vi "Dashboard Main.vi"() -> ()   [LabVIEW 2014]
uses:
  <vilib>/event_ctls.llb/eventvkey.ctl
  <vilib>/Utility/config.llb/NI_LVConfig.lvlib
  <vilib>/Rock Robotics/WPI/Dashboard/WPI_DashboardLogging Global.vi
  <vilib>/Rock Robotics/Network Tables/SD Read Number.vi
  <vilib>/Rock Robotics/Network Tables/SD Write Number.vi
  <vilib>/Utility/config.llb/Write Key (I32).vi
  <vilib>/Utility/config.llb/Write Key (String).vi
  <vilib>/Rock Robotics/Network Tables/SD Read String.vi
  <vilib>/Rock Robotics/Network Tables/SD Read Boolean.vi
  <vilib>/Rock Robotics/Network Tables/SD Write Boolean.vi
panel:
  in  "TCP":refnum<k5>
  in  "Rec Mode":enum32{"Stop", "Record", "Playback"}(radio)
  in  "Vision":u16(ring) items=["Camera Off", "USB Camera SW", "USB Camera HW", "IP Camera"]
  out "Camera IP":string
  out "Image Message":string="Timeout in Camera Communications"
  in  "Dashboard Tab":T1(tab)
  in  "Camera Guide Position":dbl(slide)=216.05839416058393 scale=0.0..320.0
  in  "Camera Settings":T2={"Frame Rate"=30, "Compression"=30, "Size"=1} {"Frame Rate" scale=1.0..30.0; "Size" items=["640x480", "320x240", "160x120"]}
  out "MotorChart R":cluster{"Numeric":dbl, "Numeric":dbl}(graph)
  out "MotorChart L":T3(graph)
  out "MotorSliders R":cluster{"MotorSlide1":dbl, "MotorSlide2":dbl} {"MotorSlide2" scale=-1.0..1.0 scale format="%#_2e"; "MotorSlide1" scale=-1.0..1.0 scale format="%#_2e"}
  out "MotorSliders L":T4 {"MotorSlide4 2" scale=0.0..14.0 scale format="%#_2e"; "MotorSlide2" scale=-1.0..1.0 scale format="%#_2e"; "MotorSlide1" scale=-1.0..1.0 scale format="%#_2e"}
  out "JS1 Z":dbl(slide) scale=-1.0..1.0 scale format="%#_2e"
  out "JS1 Graph":cluster{"X":dbl, "Y":dbl}[](graph)
  out "JS1 Buttons":T5
  out "JS2 Z":dbl(slide) scale=-1.0..1.0 scale format="%#_2e"
  out "JS2 Graph":cluster{"X":dbl, "Y":dbl}[](graph)
  out "JS2 Buttons":T5
  out "Mode":T6(ring)=enum."Auto Disabled"
  in  "DB Camera Config":bool
  out "fps":dbl format="%#.1g"
  out "Mbps":dbl format="%#.1g"
  out "Mbps 2":bool
  in  "FastAuto?":bool
  in  "AutoStackRamp":bool
  out "Current Auto":dbl
  out "Auto/String 3":string caption="DB/String 3"
  out "Auto/String 2":string caption="DB/String 2"
  out "Auto/String 1":string caption="DB/String 1"
  out "Auto/String 0":string caption="Auto"
  out "Elev. Current":dbl
  out "Can\n  Auto\n  Stack":bool
  out "PID State":T7(ring)
  in  "Training Mode Threshold":dbl=0.8
  out "Drive Mode":bool
  out "Gyro":dbl(knob) scale=0.0..360.0
  in  "Halo Sensitivity":dbl=0.7 min=0.0 max=1.0 step=0.01 format="%.2f"
  out "Encoder Left":dbl
  out "Encoder Right":dbl
  out "Training Enabled":bool
  out "Auto Stack State":T8(ring)
  out "Gripper":bool
  out "Gripper 2":bool
  out "Elev. Target":dbl
  in  "Test Slider":dbl(slide) scale=0.0..100.0 scale format="%#_3g"
  in  "On/Off":bool caption="Solenoid"
  in  "Test Name":u16(ring) items=["Select the test to run...", "Example Test", "-------------------------------", "List of tests is built in robot code.", "Replace with your own automated tests."]
  in  "Test Tree":string(tree)
  in  "Motor":cluster{"Value":dbl, "Enable":bool} {"Value" scale=-1.0..1.0 scale format="%#_3g"}
  out "Progress":T9 {"Test Progress" scale=0.0..100.0}
  in  "Rev/Fwd":cluster{"Forward":bool, "Reverse":bool}
  in  "Test Ring":u16(ring) items=["Monochrome", "Color"]
  in  "Listbox":i32(listbox)
  out "Tree":string(tree)
  out "Camera Image":T10(plugin-control)
  out "Boolean":bool
  # "Left"
  # "Front"
  # "Right"
  # "Battery"
  # "AUTO STACK"
  # "0 - TOTE+CONTAINER\n1 - DRIVESTRAIGHT FROM STARTING AREA\n2 - DRIVESTRAIGHT FROM VOLDEMORT\n3 - 2 CONTAINER + LEFT TURN\n4 - 2 CONTAINER + RIGHT TURN\n5 - STOP_ALL\n6 - TAPE MEASURE\n7 - TOTE TO FEEDER - SHORT\n8 - TOTE TO FEEDER - LONG\n9 - CAN BURGLAR"
  # "Hold BACK button on \nJoystick 1 to switch"
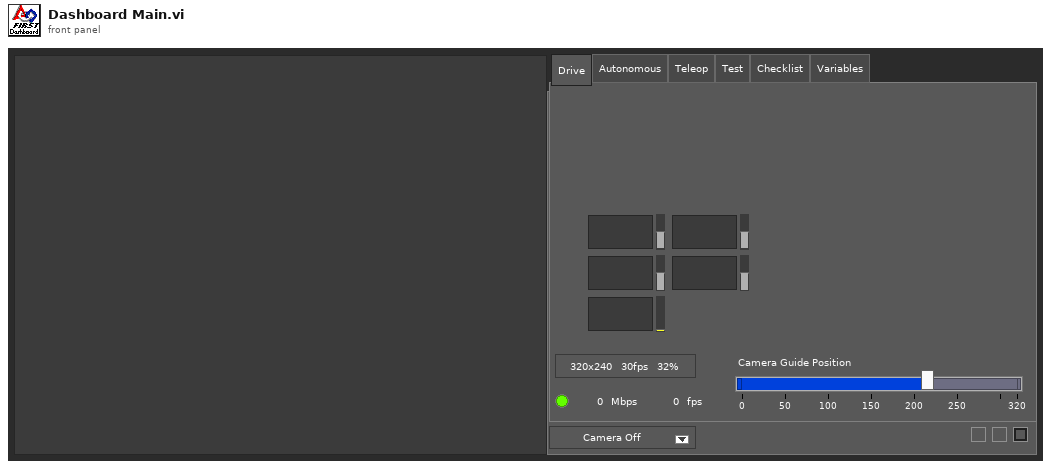
[diagram p1: front panel]
types:
  T1 = enum32{"Drive", "Autonomous", "Teleop", "Test", "Checklist", "Variables"}
  T2 = cluster{"Frame Rate":i32, "Compression":i32, "Size":u16}
  T3 = cluster{"Numeric":dbl, "Numeric":dbl, "Battery V":dbl}
  T4 = cluster{"MotorSlide1":dbl, "MotorSlide2":dbl, "MotorSlide4 2":dbl}
  T5 = cluster{bool, bool, bool, bool, bool, bool, bool, bool, bool, bool, bool, bool}
  T6 = enum8{"Tele-Op Disabled", "Tele-Op Enabled", "Auto Disabled", "Auto Enabled", "Test Disabled", "Test Enabled", "Disconnected", "No Code", "E-Stop"}
  T7 = enum16{"ResetForward", "ResetBack", "PIDControl", "ManualControl", "ZeroEncoderAndTarget", "AutoStack"}
  T8 = enum16{"Disabled", "Initialize", "CalcNewTarget", "Moving", "OpenArm", "CloseArm", "Reset"}
  T9 = cluster{"Test Progress":u8, "Test Progress Text":string}
  T10 = typedef "IMAQ Image.ctl" = refnum<image>
  T11 = enum32{"Drive", "Basic", "Custom", "Test", "Checklist", "Variables"}
  T12 = typedef "Image Type" = u32
  T13 = cluster{"Camera Image":refnum<vi>, "Dashboard Tab":refnum<vi>, "Boolean":refnum<vi>, "Vision":refnum<vi>, "Rec Mode":refnum<vi>, "Test Slider":refnum<vi>, "On/Off ":refnum<vi>, "Test Ring":refnum<vi>, "Rev/Fwd":refnum<vi>, "Test Name":refnum<vi>, "Motor":refnum<vi>, "Progress":refnum<vi>, "CheckList":refnum<vi>, "Tree":refnum<vi>, "Test Tree":refnum<vi>}
  T14 = cluster{"Error Strings":string, "Disable Counts":cluster{u16, u16}, "Rail Faults":cluster{u16, u16, u16}, "Robot IP":string, "DB Mode":u8, "Event Info":cluster{"Name":string, "Type":u8, "Number":u16, "Replay":u8}, "Camera Addr":string}
  T15 = cluster{"Storage":cluster{"Disk Free":u64, "RAM Block":u32, "RAM free":u32}, "CPU Utilization":cluster{"CPU % ISR":sgl, "CPU % Time Crit":sgl, "CPU % Timed Str":sgl, "CPU % High":sgl, "CPU % Above":sgl, "CPU % Normal":sgl, "CPU % Low":sgl}, "CAN":cluster{"% Bus Utilization":sgl, "Bus Off Cnt":u32, "TX_FIFO Full Cnt":u32, "Receive Error Cnt":u8, "Transmit Error Cnt":u8}, "HID":cluster{"HID Outputs":u32, "Rumble Low":u16, "Rumble High":u16}[]}
  T16 = cluster{"Status bits":cluster{"Test Mode":bool, "Autonomous":bool, "Enabled":bool, "Code Start":bool, "Brownout":bool, "Reserved 2":bool, "Reserved 3":bool, "E-Stop":bool}, "Code Trace":cluster{"Disabled":bool, "TeleOp":bool, "Auto":bool, "Test":bool}, "Controller Type":enum16{"unknown", "cRIO", "roboRio"}, "Code?":enum16{"unknown", "noCode", "code"}, "Battery V":dbl}
  T17 = cluster{"Control Bits":cluster{"TestMode":bool, "Autonomous":bool, "Enabled":bool, "FMS Present":bool, bool, bool, bool, "E-Stop":bool}, "Team Station ":u8, "Countdown":sgl, "Joystick Values":cluster{"Axes":dbl[], "Buttons":bool[], "POVs":i16[]}[]}
  T18 = cluster{"Axes":dbl[], "Buttons":bool[], "POVs":i16[]}[]
  T19 = cluster{"Axes":dbl[], "Buttons":bool[], "POVs":i16[]}
  T20 = cluster{"Buttons[0]":bool, "Buttons[1]":bool, "Buttons[2]":bool, "Buttons[3]":bool, "Buttons[4]":bool, "Buttons[5]":bool, "Buttons[6]":bool, "Buttons[7]":bool, "Buttons[8]":bool, "Buttons[9]":bool, "Buttons[10]":bool, "Buttons[11]":bool}
  T21 = typedef "NI_LVConfig.lvlib/Config Data RefNum.ctl" = refnum<k1>
  T22 = cluster{"Operation":enum16{"Update", "Clear"}, "Color Box":u32}[]
  T23 = typedef "eventvkey.ctl" = enum16{"ASCII", "Enter", "Return", "Shift", "Ctrl", "Alt", "Cmd", "Opt", "Caps", "NumLock", "Clear", "Break", "Up", "Down", "Left", "Right", "Insert", "Delete", "Home", "End", "PageUp", "PageDown", "Escape", "Help", "Pause", "ScrollLock", "F1", "F2", "F3", "F4", "F5", "F6", "F7", "F8", "F9", "F10", "F11", "F12", "F13", "F14", "F15", "F16", "F17", "F18", "F19", "F20", "F21", "F22", "F23", "F24", "Play", "VolumeUp", "VolumeDown", "Mute", "Two Byte Char"}
  T24 = cluster{"Image Size":bool, "Image Type":bool, "Pixel Value":bool, "ROI Information":bool, "Zoom Factor":bool}
  T25 = enum8{"Enabled", "Disabled", "Disabled and Grayed Out"}
  T26 = cluster{"Operation":enum16{"Update", "Clear"}, "Color Box":u32}
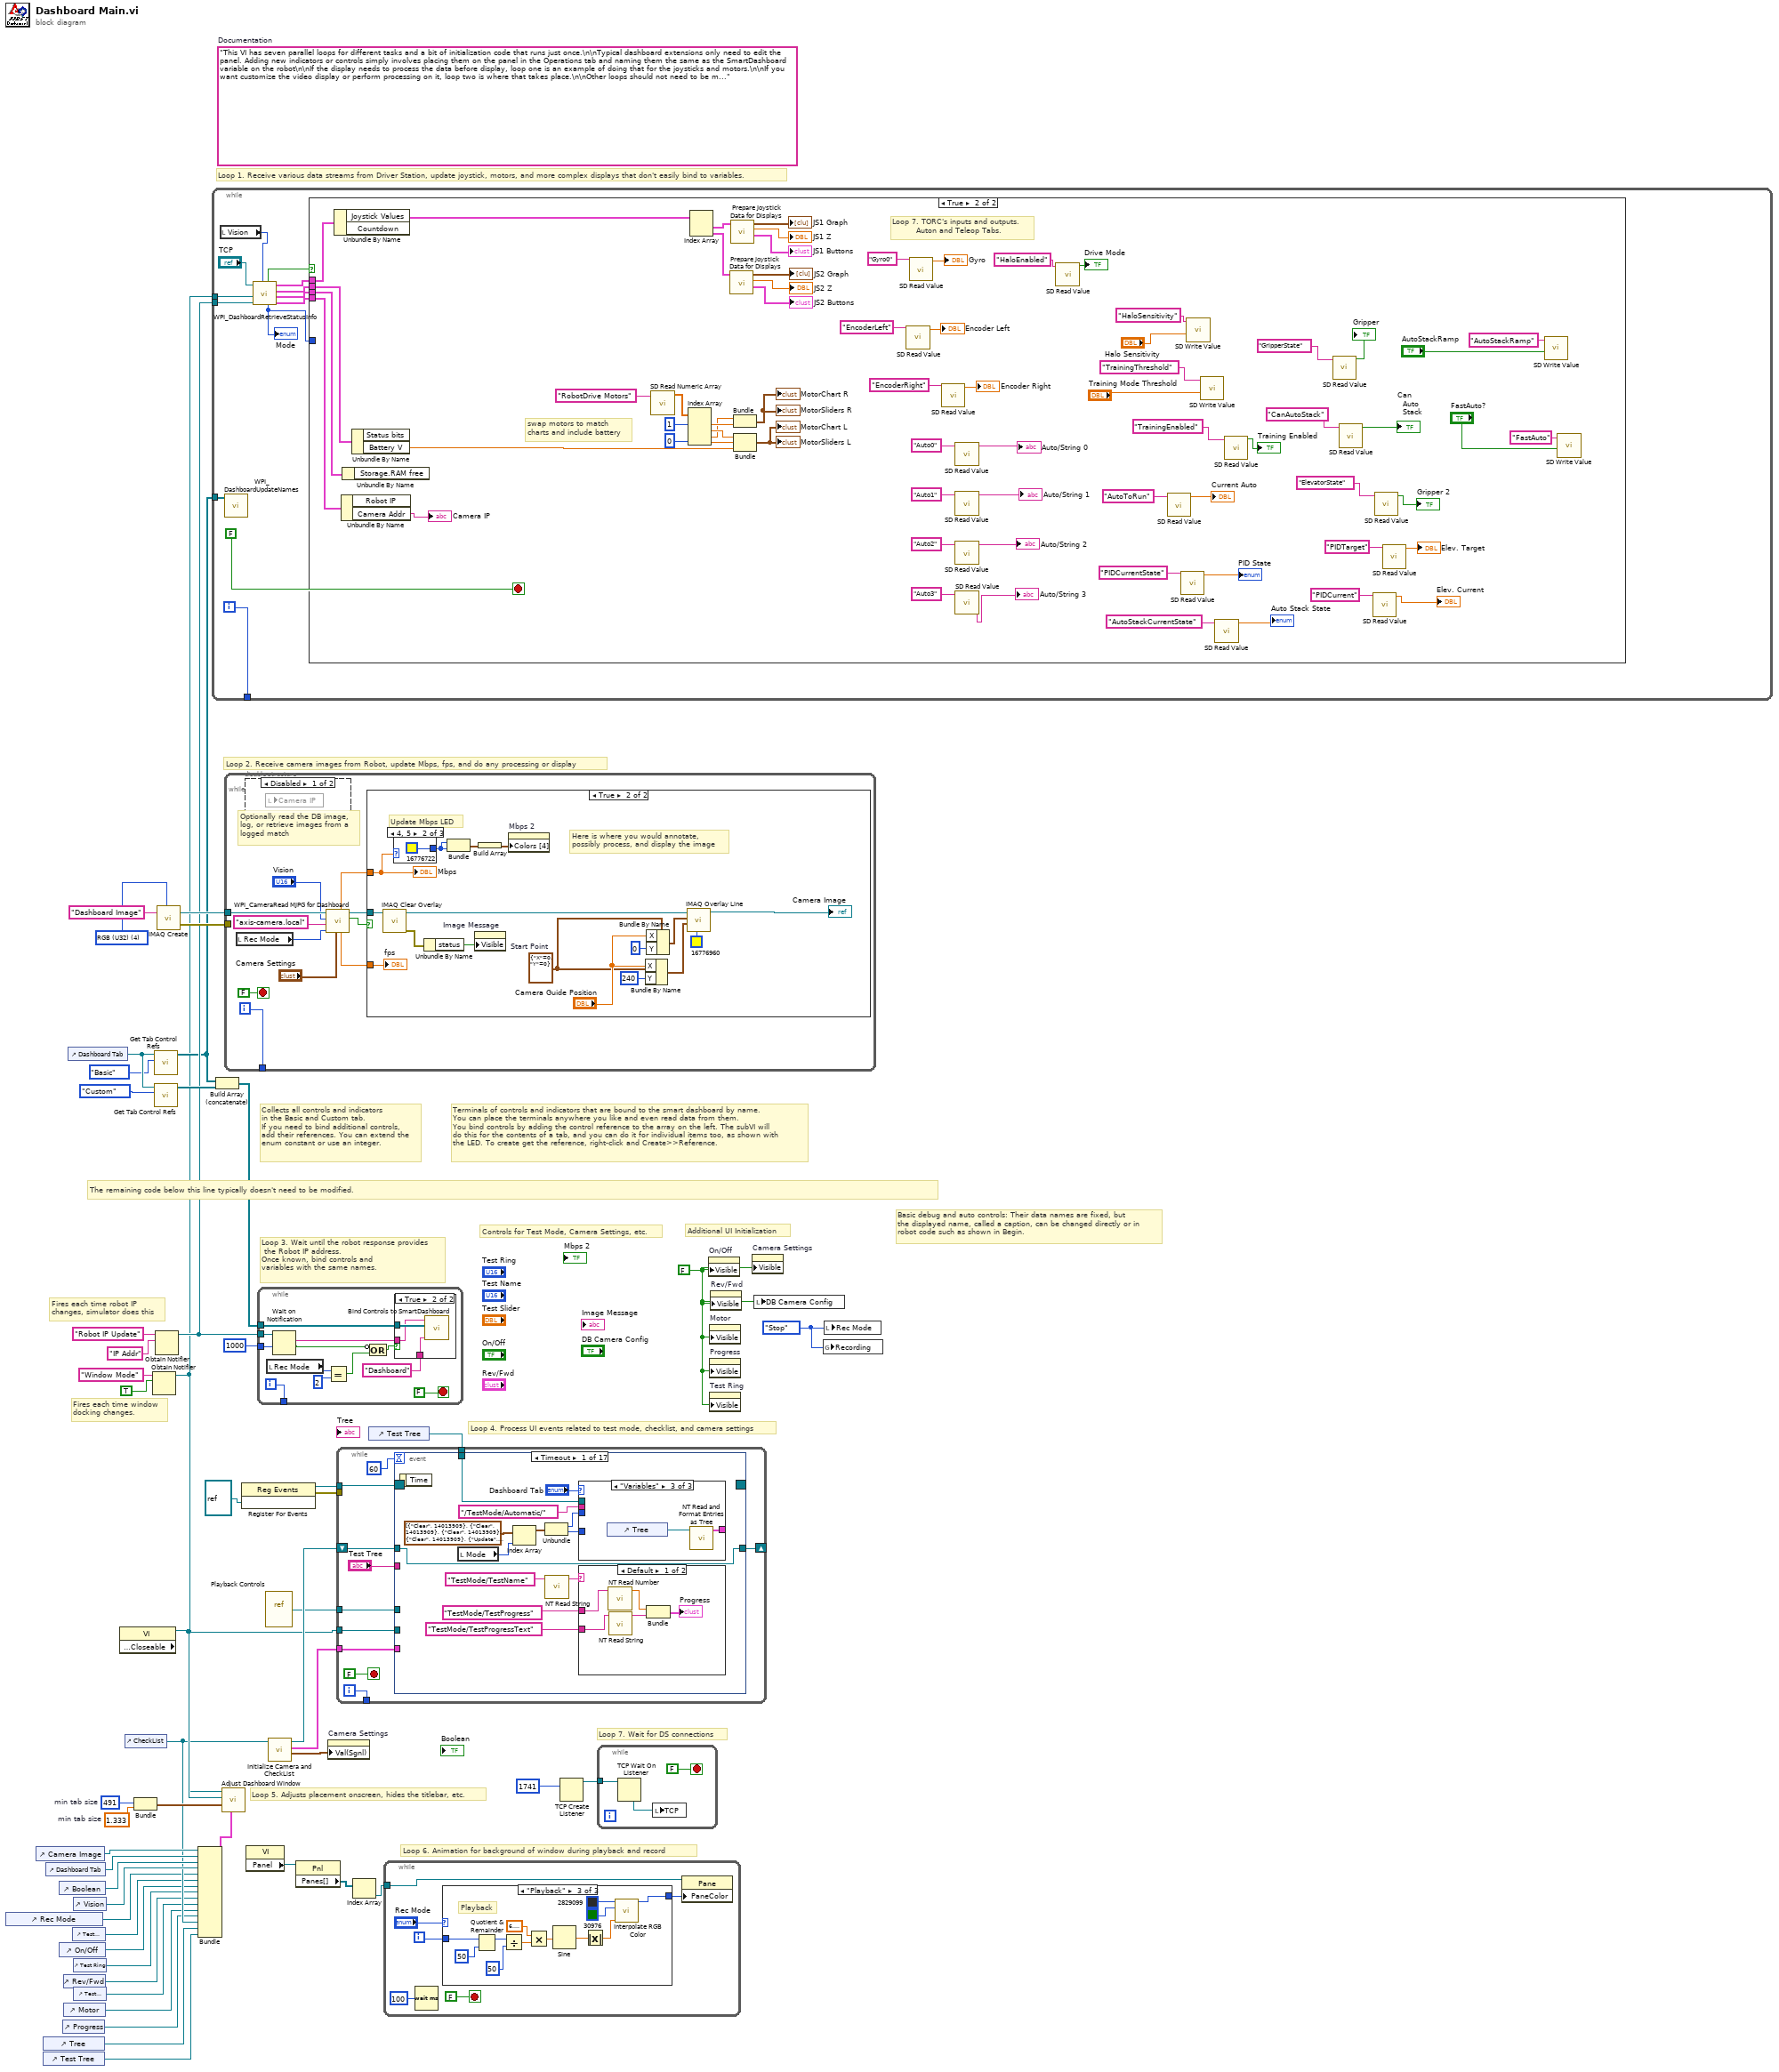
[diagram p0: block diagram]
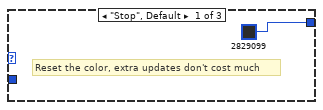
[diagram p3: hidden frame]
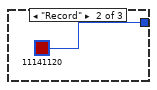
[diagram p4: hidden frame]
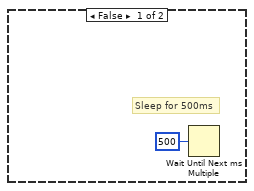
[diagram p7: hidden frame]
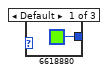
[diagram p8: hidden frame]
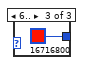
[diagram p9: hidden frame]
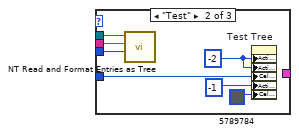
[diagram p11: hidden frame]
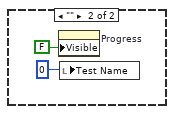
[diagram p12: hidden frame]
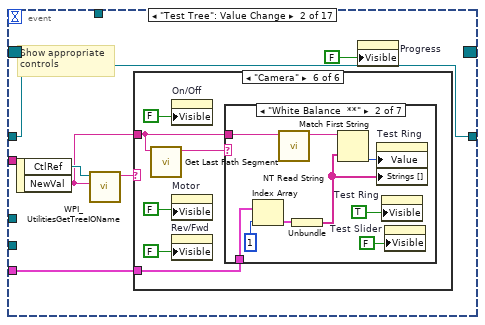
[diagram p13: hidden frame]
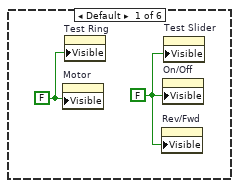
[diagram p14: hidden frame]
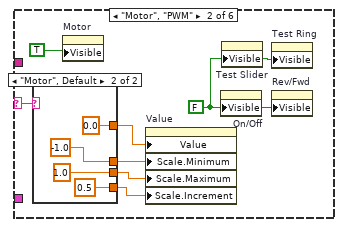
[diagram p15: hidden frame]
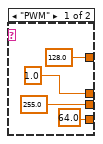
[diagram p16: hidden frame]
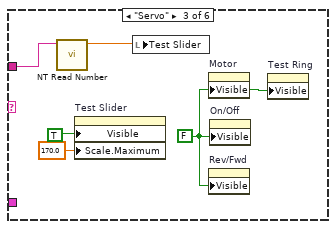
[diagram p17: hidden frame]
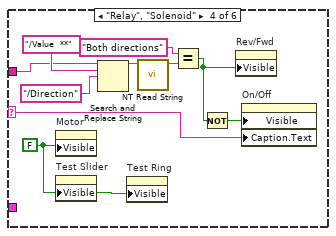
[diagram p18: hidden frame]
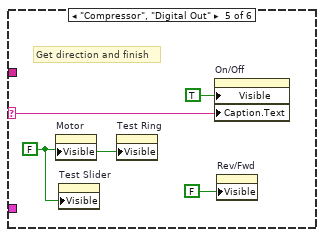
[diagram p19: hidden frame]
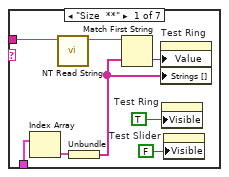
[diagram p20: hidden frame]
diagram:
  w24 = 491  # min tab size
  w23 = 1.333  # min tab size
  w32 = enum32{"Stop", "Record", "Playback"}."Stop" ("Rec Mode")
  w6 = FALSE ("Visible")
  (unwired) "This VI has seven parallel loops for different tasks and a bit of initialization code that runs just once.\n\nTypical dashboard extensions only need to edit the panel. Adding new indicators or controls simply involves placing them on the panel in the Operations tab and naming them the same as the SmartDashboard variable on the robot\n\nIf the display needs to process the data before display, loop one is an example of doing that for the joysticks and motors.\n\nIf you want customize the video display or perform processing on it, loop two is where that takes place.\n\nOther loops should not need to be modified. They are pretty standard, and document the task they perform."  # Documentation
  w52 = T12 4 items=["Grayscale (U8)", "Grayscale (I16)", "Grayscale (SGL)", "Complex (CSG)", "RGB (U32)", "HSL (U32)", "RGB (U64)"] ("Image Type")
  # "Loop 7. Wait for DS connections"
  # "Basic debug and auto controls: Their data names are fixed, but\nthe displayed name, called a caption, can be changed directly or in\nrobot code such as shown in Begin."
  # "Controls for Test Mode, Camera Settings, etc."
  # "Additional UI Initialization"
  # "Loop 6. Animation for background of window during playback and record"
  # "Fires each time robot IP\nchanges, simulator does this"
  # "Fires each time window\ndocking changes."
  # "Collects all controls and indicators\nin the Basic and Custom tab.\nIf you need to bind additional controls,\nadd their references. You can extend the\nenum constant or use an integer."
  # "The remaining code below this line typically doesn't need to be modified."
  # "Loop 4. Process UI events related to test mode, checklist, and camera settings"
  # "Terminals of controls and indicators that are bound to the smart dashboard by name.\nYou can place the terminals anywhere you like and even read data from them.\nYou bind controls by adding the control reference to the array on the left. The subVI will\ndo this for the contents of a tab, and you can do it for individual items too, as shown with\nthe LED. To create get the reference, right-click and Create>>Reference."
  # "Loop 3. Wait until the robot response provides\n the Robot IP address.\nOnce known, bind controls and\nvariables with the same names."
  # "Loop 5. Adjusts placement onscreen, hides the titlebar, etc."
  # "Loop 1. Receive various data streams from Driver Station, update joystick, motors, and more complex displays that don't easily bind to variables."
  # "Loop 2. Receive camera images from Robot, update Mbps, fps, and do any processing or display"
  n1 = control-ref of="Rec Mode"() -> (w12:refnum<vi>)
  n2 = control-ref of="Camera Image"() -> (w27:refnum<vi>)
  n3 = control-ref of="Tree"() -> (w16:refnum<vi>)
  n4 = control-ref of="Test Tree"() -> (w15:refnum<vi>)
  n5 = control-ref of="Dashboard Tab"() -> (w26:refnum<vi>)
  n6 = control-ref of="Boolean"() -> (w21:refnum<vi>)
  n7 = control-ref of="On/Off"() -> (w10:refnum<vi>)
  n8 = control-ref of="Progress"() -> (w7:refnum<vi>)
  n9 = control-ref of="Rev/Fwd"() -> (w8:refnum<vi>)
  n10 = control-ref of="Motor"() -> (w13:refnum<vi>)
  n11 = control-ref of="Dashboard Tab"() -> (w30:refnum<vi>)
  n12 = control-ref of="Test Slider"() -> (w11:refnum<vi>)
  n13 = control-ref of="Vision"() -> (w25:refnum<vi>)
  n14 = control-ref of="Test Ring"() -> (w9:refnum<vi>)
  n15 = control-ref of="Test Name"() -> (w14:refnum<vi>)
  n16 = property class="VI" props=["Front Panel.Closeable"]() -> (reference out=w31:refnum<vi>)  [unwired: 2 in, 2 out]
  n17 = control-ref of="CheckList"() -> (w17:refnum<vi>)
  n18 = Bundle("min tab size"=w24, "min tab size"=w23) -> (w22:cluster{"min tab size":i32, "min tab size":dbl})  [unwired: 1 in]
  n19 = Obtain Notifier(name (unnamed)="Window Mode", notification data type=TRUE) -> (notifier out=w3:refnum<notifier>)  [unwired: 2 in, 2 out]
  n20 = call <vilib>:"Get Tab Control Refs.vi"("Page Index"=T11."Basic" ("Dashboard Tab"), "TabControl in"=w30) -> ("ControlsOnPage"=w4:refnum<vi>[])  [unwired: 9 in]
  n21 = call <vilib>:"Get Tab Control Refs.vi"("Page Index"=T11."Custom" ("Dashboard Tab"), "TabControl in"=w30) -> ("ControlsOnPage"=w29:refnum<vi>[])  [unwired: 9 in]
  n22 = Obtain Notifier(name (unnamed)="Robot IP Update", notification data type="IP Addr" ("name (unnamed)")) -> (notifier out=w5:refnum<notifier>)  [unwired: 2 in, 2 out]
  n23 = call "IMAQ Create"("Image Name"="Dashboard Image", "Image Type"=w52) -> ("New Image"=w50:T10, "error out"=w49:errorcluster)  [unwired: 2 in, 1 out]
  n24 = Bundle("Camera Image"=w27, "Dashboard Tab"=w26, "Boolean"=w21, "Vision"=w25, "Rec Mode"=w12, "Test Slider"=w11, "On/Off"=w10, "Test Ring"=w9, "Rev/Fwd"=w8, "Test Name"=w14, "Motor"=w13, "Progress"=w7, "CheckList"=w17, "Tree"=w16, "Test Tree"=w15) -> (w18:T13)  [unwired: 1 in]
  n25 = while {
    tunnel: [w64] -> _
    tunnel: w5 -> [w63]
    tunnel: w4 -> [w62]
    tunnel: w3 -> [w59]
    i -> [w64]
    stop <- FALSE stop-if-true
    n26 = local read "Vision"() -> (w61:u16)
    n27 = call <vilib>:"WPI_DashboardUpdateNames.vi"("Controls on Tab"=w62) -> ()  [unwired: 11 in]
    n28 = call <vilib>:"WPI_DashboardRetrieveStatusInfo.vi"("Vision"=w61, "Binding Refnum"=w63, "Window Mode Notifier"=w59, "TCP Cnx"="TCP") -> ("Power and Errors"=w55:T14, "Robot Metrics"=w56:T15, "Status Info"=w57:T16, "Control Info"=w58:T17, "Robot Mode"=w54:T6, "Process?"=w53:bool)  [unwired: 2 in]
    "Mode" <- w54
    n29 = case shown="True" w53 {
      tunnel: w57 -> [_ w132]
      tunnel: w56 -> [_ w131]
      tunnel: w58 -> [_ w130]
      tunnel: w55 -> [_ w129]
      tunnel: w54 -> [_ _]
      frame False {
      }
      frame True {
        # "Loop 7. TORC's inputs and outputs.\n         Auton and Teleop Tabs."
        # "swap motors to match\ncharts and include battery"
        n30 = Unbundle By Name(w130) -> ("Joystick Values"=w117:T18)  [unwired: 1 out]
        n31 = Unbundle By Name(w129) -> ("Camera Addr"=→"Camera IP":string)  [unwired: 1 out]
        n32 = Unbundle By Name(w131) -> ()  [unwired: 1 out]
        n33 = Unbundle By Name(w132) -> ("Battery V"=w118:dbl)  [unwired: 1 out]
        n34 = call <vilib>:"SD Read Numeric Array.vi"("Name"="RobotDrive Motors") -> ("Numeric Array"=w120:dbl[])  [unwired: 8 in, 2 out]
        n35 = Index Array(array=w120, index #1=1, index #4=0) -> (element #1=w124:dbl, element #2=w125:dbl, element #3=w123:dbl, element #4=w128:dbl)  [unwired: 2 in]
        n36 = Index Array(array=w117) -> (element #1=w116:T19, element #2=w111:T19)  [unwired: 2 in]
        n37 = call "Prepare Joystick Data for Displays.vi"("Joystick Values"=w111) -> ("Buttons"=→"JS2 Buttons":T20, "Z Axis"=→"JS2 Z":dbl, "Cartesian Data"=→"JS2 Graph":cluster{"X axis":dbl, "X axis":dbl}[])  [unwired: 8 in]
        n38 = call "Prepare Joystick Data for Displays.vi"("Joystick Values"=w116) -> ("Buttons"=→"JS1 Buttons":T20, "Z Axis"=→"JS1 Z":dbl, "Cartesian Data"=→"JS1 Graph":cluster{"X axis":dbl, "X axis":dbl}[])  [unwired: 8 in]
        n39 = Bundle("Numeric"=w123, "Numeric"=w124) -> (→"MotorChart R" →"MotorSliders R":cluster{"Numeric":dbl, "Numeric":dbl})  [unwired: 1 in]
        n40 = Bundle("Numeric"=w125, "Numeric"=w128, "Battery V"=w118) -> (→"MotorChart L" →"MotorSliders L":T3)  [unwired: 1 in]
        n41 = call-poly <vilib>:"SD Read Value.vi"("Name"="EncoderLeft") -> ("Numeric"=→"Encoder Left":dbl)  [unwired: 8 in, 2 out]
        n42 = call-poly <vilib>:"SD Read Value.vi"("Name"="Gyro0") -> ("Numeric"=→"Gyro":dbl)  [unwired: 8 in, 2 out]
        n43 = call-poly <vilib>:"SD Read Value.vi"("Name"="EncoderRight") -> ("Numeric"=→"Encoder Right":dbl)  [unwired: 8 in, 2 out]
        n44 = call-poly <vilib>:"SD Read Value.vi"("Name"="Auto0") -> ("String"=→"Auto/String 0":string)  [unwired: 8 in, 2 out]
        n45 = call-poly <vilib>:"SD Read Value.vi"("Name"="Auto1") -> ("String"=→"Auto/String 1":string)  [unwired: 8 in, 2 out]
        n46 = call-poly <vilib>:"SD Read Value.vi"("Name"="Auto2") -> ("String"=→"Auto/String 2":string)  [unwired: 8 in, 2 out]
        n47 = call-poly <vilib>:"SD Read Value.vi"("Name"="Auto3") -> ("String"=→"Auto/String 3":string)  [unwired: 8 in, 2 out]
        n48 = call-poly <vilib>:"SD Read Value.vi"("Name"="HaloEnabled") -> ("Boolean"=→"Drive Mode":bool)  [unwired: 8 in, 2 out]
        n49 = call-poly <vilib>:"SD Read Value.vi"("Name"="AutoToRun") -> ("Numeric"=→"Current Auto":dbl)  [unwired: 8 in, 2 out]
        n50 = call-poly <vilib>:"SD Read Value.vi"("Name"="PIDCurrentState") -> ("Numeric"=→"PID State":dbl)  [unwired: 8 in, 2 out]
        n51 = call-poly <vilib>:"SD Write Value.vi"("Numeric"="Halo Sensitivity", "Name"="HaloSensitivity") -> ()  [unwired: 8 in, 2 out]
        n52 = call-poly <vilib>:"SD Write Value.vi"("Numeric"="Training Mode Threshold", "Name"="TrainingThreshold") -> ()  [unwired: 8 in, 2 out]
        n53 = call-poly <vilib>:"SD Read Value.vi"("Name"="AutoStackCurrentState") -> ("Numeric"=→"Auto Stack State":dbl)  [unwired: 8 in, 2 out]
        n54 = call-poly <vilib>:"SD Read Value.vi"("Name"="TrainingEnabled") -> ("Boolean"=→"Training Enabled":bool)  [unwired: 8 in, 2 out]
        n55 = call-poly <vilib>:"SD Read Value.vi"("Name"="GripperState") -> ("Boolean"=→"Gripper":bool)  [unwired: 8 in, 2 out]
        n56 = call-poly <vilib>:"SD Read Value.vi"("Name"="CanAutoStack") -> ("Boolean"=→"Can\n  Auto\n  Stack":bool)  [unwired: 8 in, 2 out]
        n57 = call-poly <vilib>:"SD Read Value.vi"("Name"="PIDCurrent") -> ("Numeric"=→"Elev. Current":dbl)  [unwired: 8 in, 2 out]
        n58 = call-poly <vilib>:"SD Read Value.vi"("Name"="ElevatorState") -> ("Boolean"=→"Gripper 2":bool)  [unwired: 8 in, 2 out]
        n59 = call-poly <vilib>:"SD Read Value.vi"("Name"="PIDTarget") -> ("Numeric"=→"Elev. Target":dbl)  [unwired: 8 in, 2 out]
        n60 = call-poly <vilib>:"SD Write Value.vi"("Boolean"="AutoStackRamp", "Name"="AutoStackRamp") -> ()  [unwired: 8 in, 2 out]
        n61 = call-poly <vilib>:"SD Write Value.vi"("Boolean"="FastAuto?", "Name"="FastAuto") -> ()  [unwired: 8 in, 2 out]
      }
    }
  }
  n62 = Build Array (concatenate)(w4, w29) -> (w28:refnum<vi>[])
  n63 = call "Adjust Dashboard Window.vi"("Sizing Refnums"=w18, "Size Constraints"=w22, "VI"=w31, "Notifier in"=w3) -> ()  [unwired: 8 in]
  n64 = while {
    tunnel: w50 -> [w141]
    tunnel: w49 -> [_]
    tunnel: [w142] -> _
    i -> [w142]
    stop <- FALSE stop-if-true
    # "Optionally read the DB image,\nlog, or retrieve images from a\nlogged match"
    n65 = local read "Rec Mode"() -> (w135:enum32{"Stop", "Record", "Playback"})
    n66 = disable-structure shown="Disabled" {
      frame Disabled {
        n67 = local read "Camera IP"() -> ()  [unwired: 1 in]
      }
      frame Enabled {
      }
    }
    n68 = call <vilib>:"WPI_CameraRead MJPG for Dashboard.vi"("Camera Settings"="Camera Settings", "Rec Mode"=w135, "Camera IP"="axis-camera.local" ("Name"), "Camera Mode"="Vision", "Refnum in"=w141) -> ("Active"=w139:bool, "Refnum out"=w140:T10, "FPS"=w138:dbl, "Bandwidth (Mbps)"=w137:dbl)  [unwired: 3 in]
    n69 = case shown="True" w139 {
      tunnel: w140 -> [_ w156]
      tunnel: w137 -> [_ w155]
      tunnel: w138 -> [_ w154]
      frame False {
        # "Sleep for 500ms"
        n70 = Wait Until Next ms Multiple(millisecond multiple=u32 500) -> ()  [unwired: 1 out]
      }
      frame True {
        w147 = cluster{"X":i32, "Y":i32} {"X"=0, "Y"=0}  # Start Point
        # "Here is where you would annotate,\npossibly process, and display the image"
        # "Update Mbps LED"
        n71 = call "IMAQ Clear Overlay"("Image"=w156) -> ("error out"=w160:errorcluster, "Image Out"=w153:T10)  [unwired: 2 in, 7 out]
        n72 = case shown="4, 5" w155 {
          tunnel: [u32 6618880 ("Color Box") u32 16776722 ("Color Box") u32 16716800 ("Color Box")] -> w157
          frame Default {
          }
          frame 4, 5 {
          }
          frame 6.. {
          }
        }
        n73 = Unbundle By Name(w160) -> ("status"=w161:bool)
        n74 = Bundle("Color Box"=w157, "Color Box"=w157) -> (w159:cluster{"Color Box":u32, "Color Box":u32})  [unwired: 1 out]
        n75 = property on="Image Message" class="Str"("Visible"=w161) -> ()  [unwired: 2 in, 2 out]
        n76 = Build Array(w159) -> (w158:cluster{"Color Box":u32, "Color Box":u32}[])
        n77 = property on="Mbps 2" class="Bool (strict)"("Colors [4]"=w158) -> ()  [unwired: 2 in, 2 out]
        n78 = Bundle By Name(cluster=w147, "X"="Camera Guide Position", "Y"=240) -> (w146:cluster{"X":i32, "Y":i32})
        n79 = Bundle By Name(cluster=w147, "X"="Camera Guide Position", "Y"=0) -> (w151:cluster{"X":i32, "Y":i32})
        n80 = call "IMAQ Overlay Line"("Color"=u32 16776960, "End Point"=w146, "Start Point"=w151, "Image"=w153) -> ("Image Out"=→"Camera Image":T10)  [unwired: 6 in, 1 out]
        "Mbps" <- w155
        "fps" <- w154
      }
    }
  }
  n81 = register-events(refnum<vi> refnum) -> (reference out=w36:refnum<event-registration>, error out=w35:errorcluster)  [unwired: 2 in]
  n82 = property class="VI"() -> ("Panel"=w39:refnum<vi>)  [unwired: 2 in, 2 out]
  n83 = while {
    tunnel: w28 -> [w176]
    tunnel: w5 -> [w174]
    tunnel: [w172] -> _
    tunnel: u32 1000 ("milliseconds to wait") -> [w171]
    i -> [w172]
    stop <- FALSE stop-if-true
    n84 = local read "Rec Mode"() -> (w167:enum32{"Stop", "Record", "Playback"})
    n85 = Wait on Notification(notifier=w174, timeout in ms (-1)=w171) -> (notification=w173:string, timed out?=w169:bool)  [unwired: 2 in, 2 out]
    n86 = Equal?(x=w167, y=u16 2 ("Rec Mode")) -> (x = y?=w168:bool)
    n87 = Compound Arithmetic op=OR(invert w169, w168) -> (w170:bool)
    n88 = case shown="True" w170 {
      tunnel: w176 -> [_ w179]
      tunnel: w173 -> [_ w178]
      tunnel: "Dashboard" -> [_ w177]
      frame False {
      }
      frame True {
        n89 = call <vilib>:"Bind Controls to SmartDashboard.vi"("Client Name"=w177, "Bound Control Refs"=w179, "Server IP Address"=w178) -> ()  [unwired: 9 in]
      }
    }
  }
  n90 = vi-ref "Playback Controls.vi"() -> (w37:refnum<vi>)
  n91 = call "Initialize Camera and CheckList.vi"("ListBox in"=w17) -> ("Cluster"=w43:cluster{"value":i32, "value":i32, "index":i32}, "Array"=w44:cluster{string[]}[], "File Refnum"=w42:T21)  [unwired: 8 in]
  n92 = property class="Pnl"(reference=w39) -> ("Panes[]"=w40:refnum<vi>[])  [unwired: 1 in, 2 out]
  n93 = property on="Camera Settings" class="Clust (strict)"("Val(Sgnl)"=w43) -> ()  [unwired: 2 in, 2 out]
  n94 = Index Array(array=w40) -> (element=w38:refnum<vi>)  [unwired: 1 in]
  n95 = control-ref of="Test Tree"() -> (w41:refnum<vi>)
  n96 = while {
    tunnel: w44 -> [w187]
    shift-right: [w186] -> _
    shift-left: w42 -> [w185]
    tunnel: [w184] -> _
    tunnel: w41 -> [w183]
    tunnel: w37 -> [w182]
    tunnel: w36 -> [w181]
    tunnel: w35 -> [_]
    tunnel: w31 -> [w180]
    i -> [w184]
    stop <- FALSE stop-if-true
    n97 = event shown="[0] Timeout" {
      selector: w181 -> [_ _ _ _ _ _ _ _ _ _ _ _ _ _ _ _ _]
      dyn-events: [_ _ _ _ _ _ _ _ _ _ _ _ _ w425 _ _ _] -> _
      timeout: u32 60 ("milliseconds to wait") -> [_ _ _ _ _ _ _ _ _ _ _ _ _ _ _ _ _]
      tunnel: w183 -> [w199 _ _ _ _ _ _ _ _ _ _ _ _ _ _ _ _]
      tunnel: "Test Tree" -> [_ _ _ _ _ _ _ _ w394 w402 w404 w408 w416 _ _ _ _]
      tunnel: w187 -> [_ w221 _ _ _ _ w358 w388 _ _ _ _ _ _ _ _ _]
      tunnel: [w195 w220 w319 w324 w332 w344 w357 w381 w393 w400 w403 w407 w415 w427 w441 w442 w452] -> w186
      tunnel: w185 -> [w195 w220 w319 w324 w332 w344 w356 w381 w393 w400 w403 w407 w415 w427 w441 w442 w452]
      tunnel: w182 -> [_ _ _ _ _ _ _ _ _ _ _ _ _ w428 _ w445 _]
      tunnel: w180 -> [_ _ _ _ _ _ _ _ _ _ _ _ _ w423 _ _ _]
      event Timeout {
        n98 = event-data() -> ()  [unwired: 1 in, 1 out]
        n99 = local read "Mode"() -> (w198:T6)
        n100 = Index Array(array=T22 [{"Operation"=enum."Clear", "Color Box"=14013909}, {"Operation"=enum."Clear", "Color Box"=14013909}, {"Operation"=enum."Clear", "Color Box"=14013909}, {"Operation"=enum."Clear", "Color Box"=14013909}, {"Operation"=enum."Update", "Color Box"=14013909}, {"Operation"=enum."Update", "Color Box"=16777215}, {"Operation"=enum."Clear", "Color Box"=14013909}, {"Operation"=enum."Clear", "Color Box"=14013909}, {"Operation"=enum."Clear", "Color Box"=14013909}], index=w198) -> (element=w193:T26)
        n101 = Unbundle(w193) -> ("Operation"=w192:enum16{"Update", "Clear"}, "Color Box"=w191:u32)
        n102 = call <vilib>:"NT Read String.vi"("Name"="TestMode/TestName") -> ("String"=w202:string)  [unwired: 9 in, 1 out]
        n103 = case shown="\"Variables\"" "Dashboard Tab" {
          tunnel: w199 -> [_ w210 _]
          tunnel: "/TestMode/Automatic/" ("Name Pattern") -> [_ w209 _]
          tunnel: w192 -> [_ w208 _]
          tunnel: [_ _ w212] -> _
          tunnel: w191 -> [_ w204 _]
          frame "Teleop", Default {
          }
          frame "Test" {
            w207 = -2 ("Active Item:Row Number")
            n104 = call <vilib>:"NT Read and Format Entries as Tree.vi"("Operation"=w208, "Name Pattern"=w209, "Tree Refnum"=w210) -> ()  [unwired: 7 in, 2 out]
            n105 = property on="Test Tree" class="Tree (strict)"("Active Item Row Number"=w207, "ActiveColNum"=w207, "CellBG"=w204, "Active Item Row Number"=-1 ("Active Item:Row Number"), "CellBG"=u32 5789784 ("Color Box")) -> ()  [unwired: 2 in, 2 out]
          }
          frame "Variables" {
            n106 = control-ref of="Tree"() -> (w211:refnum<vi>)
            n107 = call <vilib>:"NT Read and Format Entries as Tree.vi"("Tree Refnum"=w211) -> ("Formatted Strings"=w212:cluster{"Name":string, "Value":string}[])  [unwired: 9 in, 1 out]
          }
        }
        n108 = case shown="Default" w202 {
          tunnel: "TestMode/TestProgress" ("Name") -> [w214 _]
          tunnel: "TestMode/TestProgressText" ("Name") -> [w213 _]
          frame Default {
            n109 = call <vilib>:"NT Read Number.vi"("Name"=w214) -> ("Numeric"=w215:dbl)  [unwired: 9 in, 1 out]
            n110 = call <vilib>:"NT Read String.vi"("Name"=w213) -> ("String"=w216:string)  [unwired: 9 in, 1 out]
            n111 = Bundle("Numeric"=w215, "String"=w216) -> (→"Progress":cluster{"Numeric":dbl, "String":string})  [unwired: 1 in]
          }
          frame "" {
            n112 = property on="Progress" class="Clust (strict)"("Visible"=FALSE) -> ()  [unwired: 2 in, 2 out]
            n113 = local write "Test Name"(u16 0) -> ()
          }
        }
      }
      event "Test Tree": Value Change {
        # "Show appropriate\ncontrols"
        n114 = event-data() -> ("CtlRef"=w224:refnum<vi>, "NewVal"=w222:string)  [unwired: 1 in]
        n115 = call <vilib>:"WPI_UtilitiesGetTreeIOName.vi"("NewVal"=w222, "TreeControl in"=w224) -> ("I/O Name"=w225:string)  [unwired: 9 in]
        n116 = case shown="\"Camera\"" w225 {
          selector: w225 -> [_ w232 _ w250 w259 _]
          tunnel: w222 -> [_ _ w247 w249 _ w266]
          tunnel: w221 -> [_ _ _ _ _ w265]
          frame Default {
            w227 = FALSE ("Visible")
            w226 = FALSE ("Visible")
            n117 = property on="Motor" class="Clust (strict)"("Visible"=w226) -> ()  [unwired: 2 in, 2 out]
            n118 = property on="Test Ring" class="Ring (strict)"("Visible"=w226) -> ()  [unwired: 2 in, 2 out]
            n119 = property on="Rev/Fwd" class="Clust (strict)"("Visible"=w227) -> ()  [unwired: 2 in, 2 out]
            n120 = property on="On/Off" class="Bool (strict)"("Visible"=w227) -> ()  [unwired: 2 in, 2 out]
            n121 = property on="Test Slider" class="Slide (strict)"("Visible"=w227) -> ()  [unwired: 2 in, 2 out]
          }
          frame "Motor", "PWM" {
            w233 = FALSE ("Visible")
            n122 = case shown="\"Motor\", Default" w232 {
              tunnel: [1.0 ("Value") -1.0 ("Value")] -> w231
              tunnel: [255.0 ("Value") 1.0 ("Value")] -> w230
              tunnel: [128.0 ("Value") 0.0 ("Value")] -> w229
              tunnel: [64.0 ("Value") 0.5 ("Value")] -> w228
              frame "PWM" {
              }
              frame "Motor", Default {
              }
            }
            n123 = property on="Motor" class="Clust (strict)"("Visible"=TRUE) -> ()  [unwired: 2 in, 2 out]
            n124 = property on="Value" class="Slide (strict)"("Value"=w229, "Scale.Minimum"=w231, "Scale.Maximum"=w230, "Scale.Increment"=w228) -> ()  [unwired: 2 in, 2 out]
            n125 = property on="On/Off" class="Bool (strict)"("Visible"=w233) -> ()  [unwired: 2 in, 2 out]
            n126 = property on="Test Slider" class="Slide (strict)"("Visible"=w233) -> ()  [unwired: 2 in, 2 out]
            n127 = property on="Test Ring" class="Ring (strict)"("Visible"=w233) -> ()  [unwired: 2 in, 2 out]
            n128 = property on="Rev/Fwd" class="Clust (strict)"("Visible"=w233) -> ()  [unwired: 2 in, 2 out]
          }
          frame "Servo" {
            w245 = FALSE ("Visible")
            n129 = call <vilib>:"NT Read Number.vi"("Name"=w247) -> ("Numeric"=w246:dbl)  [unwired: 9 in, 1 out]
            n130 = property on="Test Slider" class="Slide (strict)"("Visible"=TRUE, "Scale.Maximum"=170.0 ("Scale.Range:Maximum")) -> ()  [unwired: 2 in, 2 out]
            n131 = local write "Test Slider"(w246) -> ()
            n132 = property on="Motor" class="Clust (strict)"("Visible"=w245) -> ()  [unwired: 2 in, 2 out]
            n133 = property on="Rev/Fwd" class="Clust (strict)"("Visible"=w245) -> ()  [unwired: 2 in, 2 out]
            n134 = property on="On/Off" class="Bool (strict)"("Visible"=w245) -> ()  [unwired: 2 in, 2 out]
            n135 = property on="Test Ring" class="Ring (strict)"("Visible"=w245) -> ()  [unwired: 2 in, 2 out]
          }
          frame "Relay", "Solenoid" {
            w248 = FALSE ("Visible")
            n136 = property on="Motor" class="Clust (strict)"("Visible"=w248) -> ()  [unwired: 2 in, 2 out]
            n137 = property on="Test Slider" class="Slide (strict)"("Visible"=w248) -> ()  [unwired: 2 in, 2 out]
            n138 = Search and Replace String(input string=w249, search string="/Value  **", replace string="/Direction") -> (result string=w255:string)  [unwired: 5 in, 3 out]
            n139 = property on="Test Ring" class="Ring (strict)"("Visible"=w248) -> ()  [unwired: 2 in, 2 out]
            n140 = call <vilib>:"NT Read String.vi"("Name"=w255) -> ("String"=w253:string)  [unwired: 9 in, 1 out]
            n141 = Equal?(x="Both directions", y=w253) -> (x = y?=w251:bool)
            n142 = Not(x=w251) -> (.not. x?=w252:bool)
            n143 = property on="Rev/Fwd" class="Clust (strict)"("Visible"=w251) -> ()  [unwired: 2 in, 2 out]
            n144 = property on="On/Off" class="Bool (strict)"("Visible"=w252, "Caption.Text"=w250) -> ()  [unwired: 2 in, 2 out]
          }
          frame "Compressor", "Digital Out" {
            w258 = FALSE ("Visible")
            # "Get direction and finish"
            n145 = property on="Motor" class="Clust (strict)"("Visible"=w258) -> ()  [unwired: 2 in, 2 out]
            n146 = property on="Test Slider" class="Slide (strict)"("Visible"=w258) -> ()  [unwired: 2 in, 2 out]
            n147 = property on="Test Ring" class="Ring (strict)"("Visible"=w258) -> ()  [unwired: 2 in, 2 out]
            n148 = property on="On/Off" class="Bool (strict)"("Visible"=TRUE, "Caption.Text"=w259) -> ()  [unwired: 2 in, 2 out]
            n149 = property on="Rev/Fwd" class="Clust (strict)"("Visible"=FALSE) -> ()  [unwired: 2 in, 2 out]
          }
          frame "Camera" {
            n150 = call <vilib>:"Get Last Path Segment.vi"("String in"=w266) -> ("String out"=w267:string)  [unwired: 10 in]
            n151 = property on="On/Off" class="Bool (strict)"("Visible"=FALSE) -> ()  [unwired: 2 in, 2 out]
            n152 = property on="Motor" class="Clust (strict)"("Visible"=FALSE) -> ()  [unwired: 2 in, 2 out]
            n153 = property on="Rev/Fwd" class="Clust (strict)"("Visible"=FALSE) -> ()  [unwired: 2 in, 2 out]
            n154 = case shown="\"White Balance  **\"" w267 {
              tunnel: w266 -> [w273 w282 w291 w300 w309 _ w315]
              tunnel: w265 -> [w271 w279 w288 w297 w306 _ _]
              frame "Size  **" {
                n155 = Index Array(array=w271) -> (element=w270:cluster{string[]})  [unwired: 1 in]
                n156 = call <vilib>:"NT Read String.vi"("Name"=w273) -> ("String"=w272:string)  [unwired: 9 in, 1 out]
                n157 = Unbundle(w270) -> (w268:string[])
                n158 = Match First String(2:w268, 3:w272) -> (0:w269:i32)  [unwired: 1 out]
                n159 = property on="Test Ring" class="Ring (strict)"("Value"=w269, "Strings []"=w268) -> ()  [unwired: 2 in, 2 out]
                n160 = property on="Test Ring" class="Ring (strict)"("Visible"=TRUE) -> ()  [unwired: 2 in, 2 out]
                n161 = property on="Test Slider" class="Slide (strict)"("Visible"=FALSE) -> ()  [unwired: 2 in, 2 out]
              }
              frame "White Balance  **" {
                n162 = Index Array(array=w279, index=1) -> (element=w280:cluster{string[]})
                n163 = call <vilib>:"NT Read String.vi"("Name"=w282) -> ("String"=w281:string)  [unwired: 9 in, 1 out]
                n164 = Unbundle(w280) -> (w277:string[])
                n165 = Match First String(2:w277, 3:w281) -> (0:w276:i32)  [unwired: 1 out]
                n166 = property on="Test Ring" class="Ring (strict)"("Value"=w276, "Strings []"=w277) -> ()  [unwired: 2 in, 2 out]
                n167 = property on="Test Ring" class="Ring (strict)"("Visible"=TRUE) -> ()  [unwired: 2 in, 2 out]
                n168 = property on="Test Slider" class="Slide (strict)"("Visible"=FALSE) -> ()  [unwired: 2 in, 2 out]
              }
              frame "Exposure  **" {
                n169 = Index Array(array=w288, index=2) -> (element=w289:cluster{string[]})
                n170 = call <vilib>:"NT Read String.vi"("Name"=w291) -> ("String"=w290:string)  [unwired: 9 in, 1 out]
                n171 = Unbundle(w289) -> (w285:string[])
                n172 = Match First String(2:w285, 3:w290) -> (0:w286:i32)  [unwired: 1 out]
                n173 = property on="Test Ring" class="Ring (strict)"("Value"=w286, "Strings []"=w285) -> ()  [unwired: 2 in, 2 out]
                n174 = property on="Test Ring" class="Ring (strict)"("Visible"=TRUE) -> ()  [unwired: 2 in, 2 out]
                n175 = property on="Test Slider" class="Slide (strict)"("Visible"=FALSE) -> ()  [unwired: 2 in, 2 out]
              }
              frame "Exposure Priority  **" {
                n176 = Index Array(array=w297, index=3) -> (element=w298:cluster{string[]})
                n177 = call <vilib>:"NT Read String.vi"("Name"=w300) -> ("String"=w299:string)  [unwired: 9 in, 1 out]
                n178 = Unbundle(w298) -> (w294:string[])
                n179 = Match First String(2:w294, 3:w299) -> (0:w295:i32)  [unwired: 1 out]
                n180 = property on="Test Ring" class="Ring (strict)"("Value"=w295, "Strings []"=w294) -> ()  [unwired: 2 in, 2 out]
                n181 = property on="Test Ring" class="Ring (strict)"("Visible"=TRUE) -> ()  [unwired: 2 in, 2 out]
                n182 = property on="Test Slider" class="Slide (strict)"("Visible"=FALSE) -> ()  [unwired: 2 in, 2 out]
              }
              frame "Color Enable  **" {
                n183 = Index Array(array=w306, index=4) -> (element=w307:cluster{string[]})
                n184 = call <vilib>:"NT Read String.vi"("Name"=w309) -> ("String"=w308:string)  [unwired: 9 in, 1 out]
                n185 = Unbundle(w307) -> (w303:string[])
                n186 = Match First String(2:w303, 3:w308) -> (0:w304:i32)  [unwired: 1 out]
                n187 = property on="Test Ring" class="Ring (strict)"("Value"=w304, "Strings []"=w303) -> ()  [unwired: 2 in, 2 out]
                n188 = property on="Test Ring" class="Ring (strict)"("Visible"=TRUE) -> ()  [unwired: 2 in, 2 out]
                n189 = property on="Test Slider" class="Slide (strict)"("Visible"=FALSE) -> ()  [unwired: 2 in, 2 out]
              }
              frame Default {
                n190 = property on="Test Ring" class="Ring (strict)"("Visible"=FALSE) -> ()  [unwired: 2 in, 2 out]
                n191 = property on="Test Slider" class="Slide (strict)"("Visible"=FALSE) -> ()  [unwired: 2 in, 2 out]
              }
              frame "Brightness  **", "Color Level  **", "Compression  **", "FPS  **", "Sharpness  **" {
                n192 = call <vilib>:"NT Read Number.vi"("Name"=w315) -> ("Numeric"=w314:dbl)  [unwired: 9 in, 1 out]
                n193 = local write "Test Slider"(w314) -> ()
                n194 = property on="Test Slider" class="Slide (strict)"("Visible"=TRUE, "Scale.Maximum"=100.0 ("Scale.Range:Maximum")) -> ()  [unwired: 2 in, 2 out]
                n195 = property on="Test Ring" class="Ring (strict)"("Visible"=FALSE) -> ()  [unwired: 2 in, 2 out]
              }
            }
          }
        }
        n196 = property on="Progress" class="Clust (strict)"("Visible"=FALSE) -> ()  [unwired: 2 in, 2 out]
      }
      event "Test Name": Mouse Enter {
        # "Populate the ring with the list of tests"
        n197 = event-data() -> ()  [unwired: 1 in, 1 out]
        n198 = call <vilib>:"NT Read String Array.vi"("Name"="TestMode/TestList") -> ("String Array"=w323:string[])  [unwired: 9 in, 1 out]
        n199 = Build Array (concatenate)("Select the test to run...", w323) -> (w322:string[])
        n200 = property on="Test Name" class="Ring (strict)"("Strings []"=w322) -> ()  [unwired: 2 in, 2 out]
      }
      event "Test Name": Value Change {
        w325 = FALSE ("Visible")
        # "Tell the robot the test name to run"
        n201 = event-data() -> ("NewVal"=w329:u16)  [unwired: 1 in]
        n202 = property on="Test Name" class="Ring (strict)"() -> ("Strings []"=w330:string[])  [unwired: 2 in, 2 out]
        n203 = local write "Progress"(T9 {"Test Progress"=0, "Test Progress Text"=""} ("Progress")) -> ()
        n204 = Index Array(array=w330, index=w329) -> (element=w328:string)
        n205 = call <vilib>:"NT Write String.vi"("String"=w328, "Name"="TestMode/TestName") -> ()  [unwired: 9 in, 1 out]
        n206 = property on="Progress" class="Clust (strict)"("Visible"=TRUE) -> ()  [unwired: 2 in, 2 out]
        n207 = property on="Motor" class="Clust (strict)"("Visible"=w325) -> ()  [unwired: 2 in, 2 out]
        n208 = property on="Test Slider" class="Slide (strict)"("Visible"=w325) -> ()  [unwired: 2 in, 2 out]
        n209 = property on="On/Off" class="Bool (strict)"("Visible"=w325) -> ()  [unwired: 2 in, 2 out]
        n210 = property on="Rev/Fwd" class="Clust (strict)"("Visible"=w325) -> ()  [unwired: 2 in, 2 out]
        n211 = property on="Test Ring" class="Ring (strict)"("Visible"=w325) -> ()  [unwired: 2 in, 2 out]
      }
      event "Listbox": Double Click {
        # "Shift clears all"
        # "Update symbols on the listbox"
        n212 = event-data() -> ("PlatMods.Shift"=w333:bool, "Row"=w335:i32)  [unwired: 1 in]
        n213 = case shown="True" w333 {
          tunnel: w335 -> [w339 _]
          tunnel: 1 -> [w338 _]
          frame False {
            n214 = property on="Listbox" class="LstBox (strict)"() -> ("Item Symbols"=w337:i32[])  [unwired: 2 in, 2 out]
            n215 = Replace Array Subset(array=w337, new element=w338, index=w339) -> (w336:i32[])
            n216 = property on="Listbox" class="LstBox (strict)"("Item Symbols"=w336) -> ()  [unwired: 2 in, 2 out]
          }
          frame True {
            w340 = 0 ("Top Row")
            n217 = property on="Listbox" class="LstBox (strict)"() -> ("Number of Rows"=w342:u32)  [unwired: 2 in, 2 out]
            n218 = Initialize Array(0, w342) -> (w341:i32[])
            n219 = property on="Listbox" class="LstBox (strict)"("Top Row"=w340, "Value"=w340, "Item Symbols"=w341) -> ()  [unwired: 2 in, 2 out]
          }
        }
      }
      event "Listbox": Key Down {
        # "Update symbols on the listbox\nLeft and right keys check and uncheck"
        n220 = event-data() -> ("VKey"=w346:T23)  [unwired: 1 in]
        n221 = case shown="\"Left\", \"Right\"" w346 {
          selector: w346 -> [w351 _]
          tunnel: eventvkey."Left" ("VKey") -> [w349 _]
          frame "Left", "Right" {
            n222 = Equal?(x=w349, y=w351) -> (x = y?=w350:bool)
            n223 = Select(t=0, s=w350, f=1) -> (s? t:f=w352:i32)
            n224 = property on="Listbox" class="LstBox (strict)"() -> ("Item Symbols"=w355:i32[])  [unwired: 2 in, 2 out]
            n225 = Replace Array Subset(array=w355, new element=w352, index="Listbox") -> (w354:i32[])
            n226 = property on="Listbox" class="LstBox (strict)"("Item Symbols"=w354) -> ()  [unwired: 2 in, 2 out]
          }
          frame Default {
          }
        }
      }
      event "DB Camera Config": Value Change {
        # "Show or hide the cluster of controls, store in ini file"
        n227 = event-data() -> ("NewVal"=w359:bool)  [unwired: 1 in]
        n228 = case shown="False" w359 {
          tunnel: w358 -> [w368 _]
          tunnel: [w361 w379] -> w357
          tunnel: w356 -> [w360 w379]
          frame False {
            w375 = "Camera"
            w378 = FALSE ("Visible")
            n229 = local read "Camera Settings"() -> (w367:T2)
            n230 = Index Array(array=w368) -> (element=w371:cluster{string[]})  [unwired: 1 in]
            n231 = Unbundle(w367) -> ("Frame Rate"=w366:i32, "Compression"=w365:i32, "Size"=w369:u16)
            n232 = Unbundle(w371) -> (w370:string[])
            n233 = Index Array(array=w370, index=w369) -> (element=w364:string)
            n234 = call-poly <vilib>:"Write Key.vi"("section"=w375, "value"=w364, "key"="Size", "refnum"=w360) -> ("refnum out"=w377:T21)  [unwired: 2 in, 5 out]
            n235 = call-poly <vilib>:"Write Key.vi"("section"=w375, "value"=w366, "key"="FrameRate", "refnum"=w377) -> ("refnum out"=w376:T21)  [unwired: 1 in, 6 out]
            n236 = property on="Camera Settings" class="Clust (strict)"("Visible"=w378) -> ()  [unwired: 2 in, 2 out]
            n237 = local write "DB Camera Config"(w378) -> ()
            n238 = call-poly <vilib>:"Write Key.vi"("section"=w375, "value"=w365, "key"="Compression", "refnum"=w376) -> ("refnum out"=w362:T21)  [unwired: 1 in, 6 out]
            n239 = call <vilib>:"Close Config Data.vi"("refnum"=w362) -> ("file path"=w363:path)  [unwired: 2 in, 8 out]
            n240 = call <vilib>:"Open Config Data.vi"("configuration file path"=w363) -> ("refnum"=w361:T21)  [unwired: 8 in, 2 out]
          }
          frame True {
            n241 = property on="Camera Settings" class="Clust (strict)"("Visible"=TRUE) -> ()  [unwired: 2 in, 2 out]
          }
        }
      }
      event "Camera Settings": Value Change {
        # "Update summary string when any elements of DB camera change"
        n242 = event-data() -> ("NewVal"=w392:T2)  [unwired: 1 in]
        n243 = Index Array(array=w388) -> (element=w387:cluster{string[]})  [unwired: 1 in]
        n244 = Unbundle(w392) -> ("Frame Rate"=w383:i32, "Compression"=w382:i32, "Size"=w385:u16)
        n245 = Unbundle(w387) -> (w386:string[])
        n246 = Index Array(array=w386, index=w385) -> (element=w384:string)
        n247 = Format Into String(format string="%s   %dfps   %d%%", w384, w383, w382) -> (resulting string=w389:string)  [unwired: 2 in, 1 out]
        n248 = Build Array(w389) -> (w390:string[])
        n249 = property on="DB Camera Config" class="Bool (strict)"("Strings [4]"=w390) -> ()  [unwired: 2 in, 2 out]
      }
      event "Motor.Enable": Value Change {
        # "When the test mode otor enable helper is set, update that\ntree row item's value"
        n250 = event-data() -> ("NewVal"=w398:bool)  [unwired: 1 in]
        n251 = Unbundle("Motor") -> ("Value"=w397:dbl)  [unwired: 1 out]
        n252 = Select(t=w397, s=w398, f=0.0) -> (s? t:f=w395:dbl)
        n253 = call <vilib>:"NT Write Number.vi"("Numeric"=w395, "Name"=w394) -> ()  [unwired: 9 in, 1 out]
      }
      event "Test Slider": Value Change {
        # "When the test mode slider helper is set, update that\ntree row item's value"
        n254 = event-data() -> ("NewVal"=w401:dbl)  [unwired: 1 in]
        n255 = call <vilib>:"NT Write Number.vi"("Numeric"=w401, "Name"=w402) -> ()  [unwired: 9 in, 1 out]
      }
      event "On/Off": Value Change {
        # "When the test mode on/off helper value is set, update that\ntree row item's value"
        n256 = event-data() -> ("NewVal"=w406:bool)  [unwired: 1 in]
        n257 = Boolean To (0,1)(Boolean=w406) -> (0, 1=w405:i16)
        n258 = call <vilib>:"NT Write Number.vi"("Numeric"=w405, "Name"=w404) -> ()  [unwired: 9 in, 1 out]
      }
      event "Rev/Fwd": Value Change {
        # "When the test mode helper value for relays is set, update that\ntree row item's value"
        n259 = event-data() -> ("NewVal.Forward"=w414:bool, "NewVal.Reverse"=w413:bool)  [unwired: 1 in]
        n260 = Boolean To (0,1)(Boolean=w414) -> (0, 1=w410:i16)
        n261 = Boolean To (0,1)(Boolean=w413) -> (0, 1=w412:i16)
        n262 = Negate(x=w412) -> (-x=w411:i16)
        n263 = Add(x=w410, y=w411) -> (x+y=w409:i16)
        n264 = call <vilib>:"NT Write Number.vi"("Numeric"=w409, "Name"=w408) -> ()  [unwired: 9 in, 1 out]
      }
      event "Test Ring": Value Change {
        # "When a test mode helper value is selected from the ring,\nset the tree item's variable to the string value"
        n265 = event-data() -> ("NewVal"=w418:u16)  [unwired: 1 in]
        n266 = property on="Test Ring" class="Ring (strict)"() -> ("Strings []"=w419:string[])  [unwired: 2 in, 2 out]
        n267 = Index Array(array=w419, index=w418) -> (element=w417:string)
        n268 = call <vilib>:"NT Write String.vi"("String"=w417, "Name"=w416) -> ()  [unwired: 9 in, 1 out]
      }
      event "Rec Mode": Value Change {
        # "Update globals for recording mode and path to read log from.\nClear when logging and let NetworkTables set path for vision to\nuse."
        n269 = event-data() -> ("NewVal"=w429:enum32{"Stop", "Record", "Playback"})  [unwired: 1 in]
        n270 = global write "WPI_DashboardLogging Global.vi" "Logging Filename"(path "") -> ()
        n271 = case shown="\"Playback\"" w429 {
          tunnel: w428 -> [_ w431 w439]
          tunnel: [_ _ w438] -> w425
          tunnel: [_ _ w437] -> _
          tunnel: w423 -> [_ _ w435]
          tunnel: cluster{i32, i32} {-250, 170} -> [_ _ w434]
          tunnel: [_ _ T24 {"Image Size"=TRUE, "Image Type"=TRUE, "Pixel Value"=TRUE, "ROI Information"=TRUE, "Zoom Factor"=FALSE} ("Image Information Shown:All Elements")] -> w421
          tunnel: [_ _ TRUE ("Zoom Factor")] -> w420
          frame Default {
          }
          frame "Stop", "Record" {
            # "Place Window too"
            n272 = invoke class="VI" method="FP.Close"(reference=w431) -> (reference out=w430:refnum<vi>)  [unwired: 2 in, 2 out]
            n273 = invoke class="VI" method="Abort VI"(reference=w430) -> ()  [unwired: 2 in, 3 out]
          }
          frame "Playback" {
            n274 = call "Open Playback Panel.vi"("Offset"=w434, "DB VI Ref"=w435, "Playback in"=w439) -> ("Playback out"=w436:refnum<vi>)  [unwired: 8 in]
            n275 = register-events(w436) -> (reference out=w438:refnum<event-registration>, error out=w437:errorcluster)  [unwired: 2 in]
          }
        }
        n276 = global write "WPI_DashboardLogging Global.vi" "Recording"(w429) -> ()
        n277 = property on="Camera Image" class="ImageControl"("Image Information Shown"=w421, "Image Information Visible"=w420) -> ()  [unwired: 2 in, 2 out]
        n278 = call <vilib>:"WPI_DashboardNT Log FieldName Cache.vi"("Operation"=enum16{"Lookup/Add", "Index", "Clear"}."Clear") -> ()  [unwired: 8 in, 3 out]
      }
      event Panel Close {
        w440 = enum32{"Stop", "Record", "Playback"}."Stop" ("Rec Mode")
        # "Playback window has been closed, abort"
        n279 = event-data() -> ()  [unwired: 1 in, 4 out]
        n280 = local write "Rec Mode"(w440) -> ()
        n281 = global write "WPI_DashboardLogging Global.vi" "Recording"(w440) -> ()
      }
      event Panel Close {
        # "Abort playback window and ourself"
        n282 = event-data() -> ()  [unwired: 1 in, 4 out]
        n283 = invoke class="VI" method="FP.Close"(reference=w445) -> (reference out=w444:refnum<vi>)  [unwired: 2 in, 2 out]
        n284 = invoke class="VI" method="Abort VI"(reference=w444) -> (error out=w443:errorcluster)  [unwired: 2 in, 2 out]
        n285 = invoke class="VI" method="Abort VI"(error in=w443) -> ()  [unwired: 2 in, 3 out]
      }
      event "Vision": Value Change {
        # "Enable/Disable Compression slider.\nHW USB is hard-coded into the camera"
        n286 = event-data() -> ("NewVal"=w451:u16)  [unwired: 1 in]
        n287 = Equal?(x=w451, y=u32 2 ("milliseconds to wait")) -> (x = y?=w449:bool)
        n288 = Select(t=T25."Disabled and Grayed Out" ("Disabled"), s=w449, f=T25."Enabled" ("Disabled")) -> (s? t:f=w446:T25)
        n289 = property on="Compression" class="Slide (strict)"("DisabledEnum"=w446) -> ()  [unwired: 2 in, 2 out]
      }
    }
  }
  n290 = while {
    tunnel: w38 -> [w454]
    i -> [w457]
    stop <- FALSE stop-if-true
    n291 = Wait (ms)(milliseconds to wait=u32 100) -> ()  [unwired: 1 out]
    n292 = case shown="\"Playback\"" "Rec Mode" {
      tunnel: w457 -> [_ _ w472]
      tunnel: [u32 2829099 ("Base Color") u32 11141120 ("Target Color") w461] -> w453
      frame "Stop", Default {
        # "Reset the color, extra updates don't cost much"
      }
      frame "Record" {
      }
      frame "Playback" {
        # "Playback"
        n293 = Quotient & Remainder(x=w472, y=u32 50 ("milliseconds to wait")) -> (x-y*floor(x/y)=w468:u32)  [unwired: 1 out]
        n294 = Divide(x=w468, y=u32 50 ("milliseconds to wait")) -> (x/y=w465:dbl)
        n295 = Multiply(x=6.283185307179586, y=w465) -> (x*y=w470:dbl)
        n296 = Sine(x=w470) -> (sin(x)=w469:dbl)
        n297 = Absolute Value(x=w469) -> (abs(x)=w462:dbl)
        n298 = call "Interpolate RGB Color.vi"("Proportion"=w462, "Target Color"=u32 30976, "Base Color"=u32 2829099) -> ("Result Color"=w461:u32)  [unwired: 8 in]
      }
    }
    n299 = property class="Pane"(reference=w454, "PaneColor"=w453) -> ()  [unwired: 1 in, 2 out]
  }
  n300 = TCP Create Listener(10:u16 1741 ("timeout ms (25000)")) -> (3:w1:refnum<k5>)  [unwired: 4 in, 2 out]
  n301 = while {
    tunnel: w1 -> [w474]
    stop <- FALSE stop-if-true
    n302 = TCP Wait On Listener(11:w474) -> (4:w473:refnum<k5>)  [unwired: 3 in, 4 out]
    n303 = local write "TCP"(w473) -> ()
  }
  n304 = property on="On/Off" class="Bool (strict)"("Visible"=w6) -> ()  [unwired: 2 in, 2 out]
  n305 = property on="Motor" class="Clust (strict)"("Visible"=w6) -> ()  [unwired: 2 in, 2 out]
  n306 = property on="Progress" class="Clust (strict)"("Visible"=w6) -> ()  [unwired: 2 in, 2 out]
  n307 = property on="Test Ring" class="Ring (strict)"("Visible"=w6) -> ()  [unwired: 2 in, 2 out]
  n308 = property on="Rev/Fwd" class="Clust (strict)"("Visible"=w6) -> ()  [unwired: 2 in, 2 out]
  n309 = property on="Camera Settings" class="Clust (strict)"("Visible"=w6) -> ()  [unwired: 2 in, 2 out]
  n310 = local write "DB Camera Config"(w6) -> ()
  n311 = global write "WPI_DashboardLogging Global.vi" "Recording"(w32) -> ()
  n312 = local write "Rec Mode"(w32) -> ()
